vi "Post Launch Initialize.vi"(8 "error in":errorcluster, 9 "Active Device":refnum<vi>, 10 "GUI Reference":refnum<vi>, 11 "Instruments in":refnum<class "Instruments.lvclass">) -> (0 "error out":errorcluster, 3 "Instruments out":refnum<class "Instruments.lvclass">, 4 "Registered Events":T1, 6 "Self Enqueuer":refnum<class "Message Enqueuer.lvclass">)   [LabVIEW 2023, in "Instruments.lvlib" / "Instruments.lvclass"]
uses:
  Library/Instruments.lvclass
  C:/Users/Public/Documents/Development/builds/Engine/Engine.lvlibp/Project/Engine.lvclass
  builds/Engine/Panel.lvlibp/Panel Helper/Panel Events.ctl
  builds/Engine/Panel.lvlibp/Panel Helper/Events.ctl
  builds/Engine/Engine.lvlibp/Custom Controls/Engine Events.ctl
  builds/Engine/Engine.lvlibp/Custom Controls/System Events.ctl
  builds/Engine/Engine.lvlibp/Custom Controls/System Status.ctl
  builds/Engine/Engine.lvlibp/Custom Controls/Manual Events.ctl
  builds/Engine/Engine.lvlibp/Custom Controls/UUT_Events.ctl
  builds/Engine/Engine.lvlibp/Custom Controls/Interface Events.ctl
  builds/Engine/Actor Framework.lvlibp/1abvi3w/vi.lib/ActorFramework/Message Enqueuer/Message Enqueuer.lvclass
  Library/Instruments.lvclass/Instruments.ctl
  Private/Accessors/Write Active Device.vi
  builds/Engine/Engine.lvlibp/Accessors/Write VI_Ref.vi
  builds/Engine/Engine.lvlibp/Accessors/Read Events.vi
  builds/Engine/Panel Manager.lvlibp/Panel Actor/Panel Actor.lvclass
  C:/Users/Public/Documents/Development/builds/Engine/Panel Manager.lvlibp/Panel Actor/Panel Actor.lvclass
  builds/Engine/Panel.lvlibp/Panel Helper/Panel Helper.lvclass
  builds/Engine/Engine.lvlibp/Project/Engine.lvclass
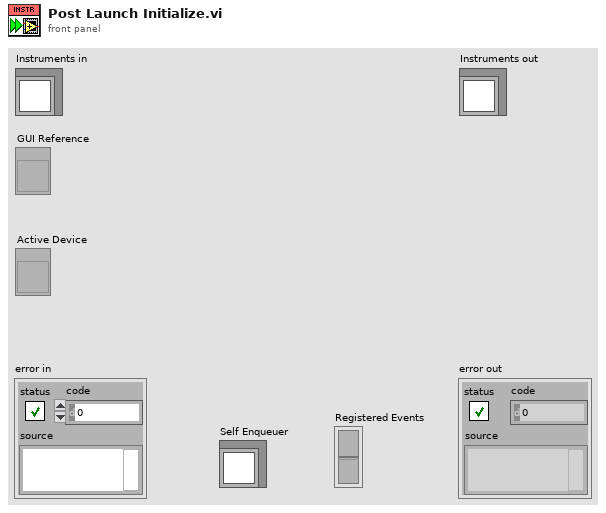
[diagram p1: front panel]
types:
  T1 = cluster{"Pnl Actor":refnum<event-registration>, "Event Registration Refnum":refnum<event-registration>}
  T2 = typedef "Engine.lvlibp/Engine.lvclass/Engine Events.ctl" = cluster{"System Event":T3, "Manual":T4, "UUT":T5, "Interface Events":T6}
  T3 = typedef "Engine.lvlibp/Engine.lvclass/System Events.ctl" = cluster{"Fault Event":refnum<user-event>, "SystemStatus Event":refnum<user-event>, "Automation":refnum<user-event>}
  T4 = typedef "Engine.lvlibp/Engine.lvclass/Manual Events.ctl" = cluster{"QuickStart Event":refnum<user-event>, "SafeBTE Event":refnum<user-event>, "TogglePower Event":refnum<user-event>, "Change Instrument Event":refnum<user-event>, "Toggle Launch Event":refnum<user-event>, "UUTSupply":refnum<user-event>}
  T5 = typedef "Engine.lvlibp/Engine.lvclass/UUT_Events.ctl" = cluster{"UUT_Name":refnum<user-event>, "Test_Name":refnum<user-event>, "Test_Operator":refnum<user-event>, "Test_Witness":refnum<user-event>, "Pedigree_Event":refnum<user-event>}
  T6 = typedef "Engine.lvlibp/Engine.lvclass/Interface Events.ctl" = cluster{"Interface_Command":refnum<user-event>, "Telemetry_Descriptor":refnum<user-event>, "AsynchTLM_Descriptor":refnum<user-event>}
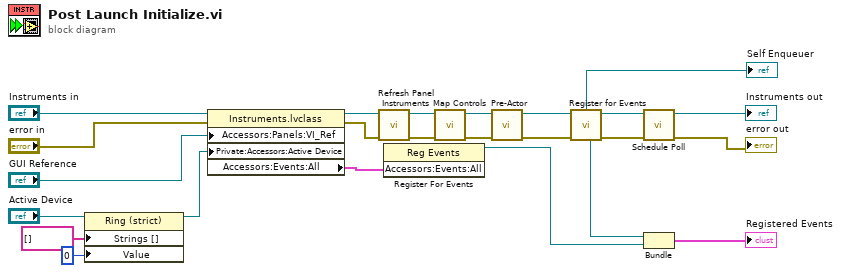
[diagram p0: block diagram]
diagram:
  n1 = property class="Ring (strict)"(reference="Active Device", "Strings []"=string[] [], "Value"=u16 0) -> (reference out=w20:refnum<vi>)  [unwired: 1 in, 1 out]
  n2 = property class="Instruments.lvclass"(reference="Instruments in", error in="error in", "Accessors:Panels:VI_Ref"="GUI Reference", "Private:Accessors:Active Device"=w20) -> (reference out=w10:refnum<class "Instruments.lvclass">, error out=w9:errorcluster, "Accessors:Events:All"=w14:T2)
  n3 = call "Refresh Panel Instruments.vi"("error in"=w9, "Instruments in"=w10) -> ("error out"=w3:errorcluster, "Instruments out"=w4:refnum<class "Instruments.lvclass">)  [unwired: 8 in]
  n4 = register-events(w14) -> (reference out=w13:refnum<event-registration>)  [unwired: 2 in, 1 out]
  n5 = call "Map Controls.vi"("error in"=w3, "Instruments in"=w4) -> ("error out"=w1:errorcluster, "Instruments out"=w2:refnum<class "Instruments.lvclass">)  [unwired: 8 in]
  n6 = call-dynamic "Pre-Actor.vi"("error in (no error)"=w1, "Instruments in"=w2) -> ("error out"=w16:errorcluster, "Instruments out"=w17:refnum<class "Instruments.lvclass">)  [unwired: 8 in]
  n7 = call "Register for Events.vi"("Error In"=w16, "Panel Actor in"=w17) -> ("Error Out"=w7:errorcluster, "Panel Actor out"=w8:refnum<class "Instruments.lvclass">, "Pnl Actor"=w15:refnum<event-registration>, "Self Enqueuer"=→"Self Enqueuer":refnum<class "Message Enqueuer.lvclass">)  [unwired: 6 in]
  n8 = call "Schedule Poll.vi"("error in"=w7, "Instruments in"=w8) -> ("error out"=→"error out":errorcluster, "Instruments out"=→"Instruments out":refnum<class "Instruments.lvclass">)  [unwired: 8 in]
  n9 = Bundle("Pnl Actor"=w15, "Event Registration Refnum"=w13) -> (→"Registered Events":T1)  [unwired: 1 in]
